vi "Model Config.vi"() -> ()   [LabVIEW 2015]
panel:
  out "error out":errorcluster
  in  "Exit":bool
  in  "Save":bool
  in  "Config Data":T1(array[cluster])
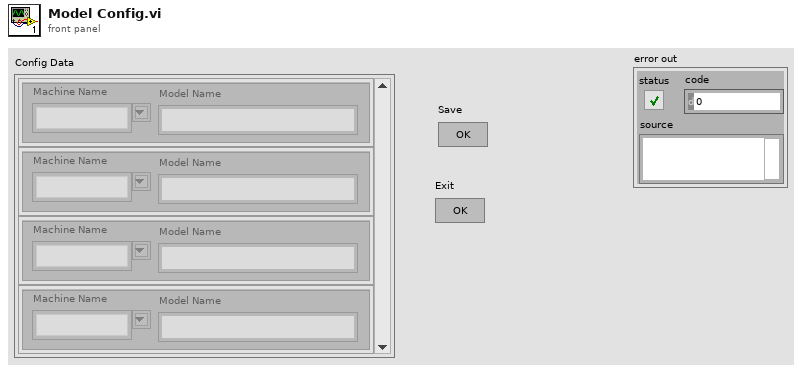
[diagram p1: front panel]
types:
  T1 = cluster{"Machine Name":string, "Model Name":string}[]
  T2 = cluster{"Machine Name":string, "Model Name":string}
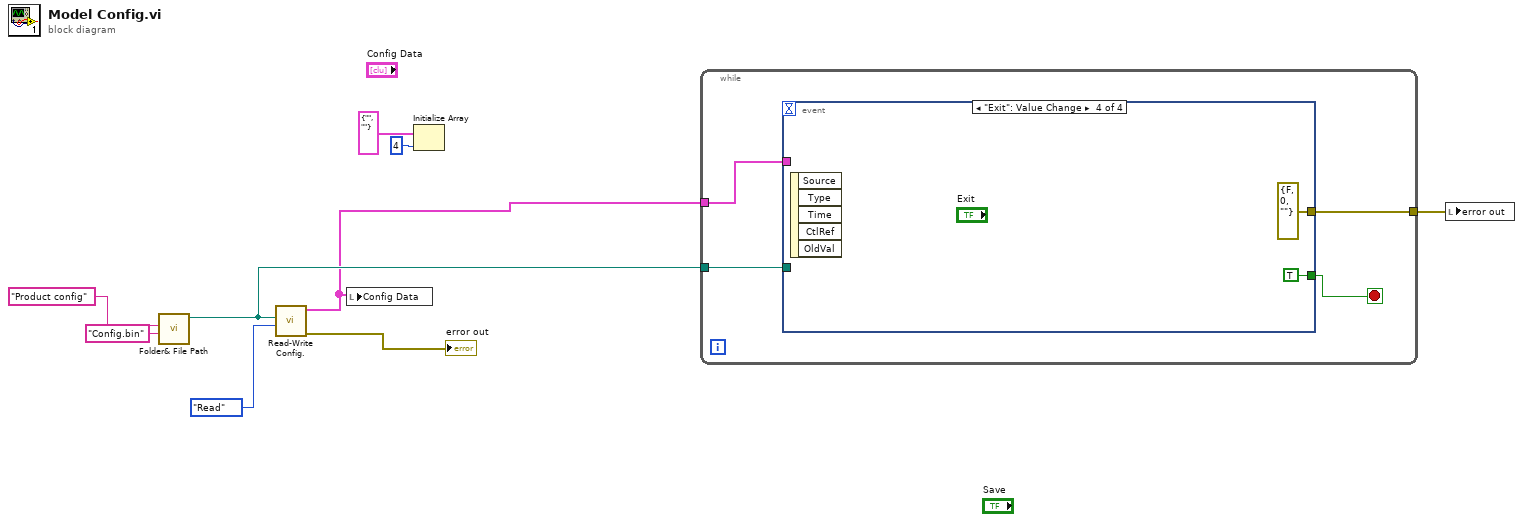
[diagram p0: block diagram]
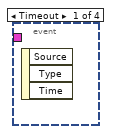
[diagram p2: hidden frame]
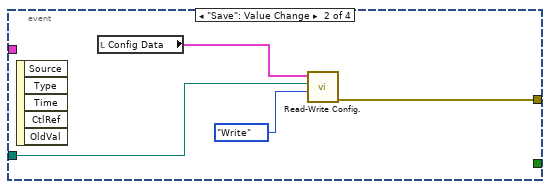
[diagram p3: hidden frame]
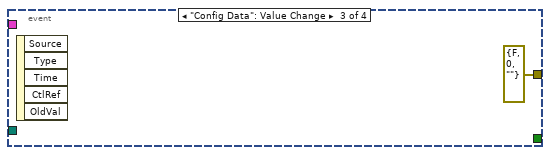
[diagram p4: hidden frame]
diagram:
  n1 = call "Folder& File Path.vi"("File Name"="Config.bin", "Folder Name"="Product config") -> ("appended path"=w5:path)  [unwired: 9 in]
  n2 = call "Read-Write Config..vi"("Enum"=enum16{"Write", "Read"}."Read", "file path (use dialog)"=w5) -> ("error out"=→"error out":errorcluster, "Read Data"=w1:T1)  [unwired: 8 in]
  n3 = local write "Config Data"(w1) -> ()
  n4 = Initialize Array(T2 {"Machine Name"="", "Model Name"=""} ("element"), 4 ("dimension size")) -> ()  [unwired: 1 out]
  n5 = while {
    tunnel: w1 -> [w12]
    tunnel: w5 -> [w11]
    tunnel: [w10] -> w4
    stop <- w13 stop-if-true
    n6 = event shown="[3] \"Exit\": Value Change" {
      selector: _ -> [_ _ _ _]
      dyn-events: _ -> [_ _ _ _]
      timeout: _ -> [_ _ _ _]
      tunnel: [_ _ _ TRUE ("Exit")] -> w13
      tunnel: w12 -> [_ _ _ _]
      tunnel: w11 -> [_ w16 _ _]
      tunnel: [_ w14 errorcluster {"status"=FALSE, "code"=0, "source"=""} ("error out") errorcluster {"status"=FALSE, "code"=0, "source"=""} ("error out")] -> w10
      event Timeout {
        n7 = event-data() -> ()  [unwired: 1 in, 3 out]
      }
      event "Save": Value Change {
        n8 = event-data() -> ()  [unwired: 1 in, 5 out]
        n9 = local read "Config Data"() -> (w15:T1)
        n10 = call "Read-Write Config..vi"("Enum"=enum16{"Write", "Read"}."Write", "file path (use dialog)"=w16, "Write Data"=w15) -> ("error out"=w14:errorcluster)  [unwired: 7 in, 1 out]
      }
      event "Config Data": Value Change {
        n11 = event-data() -> ()  [unwired: 1 in, 5 out]
      }
      event "Exit": Value Change {
        n12 = event-data() -> ()  [unwired: 1 in, 5 out]
      }
    }
  }
  n13 = local write "error out"(w4) -> ()
